vi "cycloid_text_file_generator.vi"() -> ()   [LabVIEW 2025]
panel:
  out "?":path
  out "cycle time triangle":dbl min=0.0 step=0.01
  out "Total # points triangle":i32 min=0 step=1
  out "Total Time triangle":dbl min=0.0 step=0.01
  out "Total time for one cycle Triangle":dbl min=0.0 step=0.01
  out "A3":dbl min=0.0 step=0.01
  out "f_rise":dbl min=0.0 step=0.01
  out "Trs":dbl min=0.0 step=0.01
  out "Instantaneous Flyback Time Sawtooth":dbl min=0.0 step=0.01
  out "cycle time sawtooth":dbl min=0.0 step=0.01
  out "Total Time sawtooth":dbl min=0.0 step=0.01
  out "Total # points sawtooth":i32 min=0 step=1
  in  "Number of cycles":i32=1
  in  "Sample rate":i32=5000
  out "Total time for one cycle Sawtooth":dbl min=0.0 step=0.01
  out "A0 Offset By Position Error":dbl min=0.0 step=0.01
  out "A1 Offset By Position Error":dbl min=0.0 step=0.01
  out "Position error":dbl min=0.0 step=0.01
  out "A2":dbl min=0.0 step=0.01
  out "W":dbl=28.0 min=0.0 step=0.01
  in  "T":dbl=0.01 min=0.0 step=0.001
  out "Tf":dbl=-0.44999999999999996 min=0.0 step=0.01
  in  "Tracking Delay":dbl=1e-05 min=0.0 step=1e-05
  out "A0":dbl
  in  "Cycloid selector":u16(ring) items=["Triangle", "Sawtooth"]
  in  "OK Button":bool
  in  "stop button":bool
  out "XY Graph":cluster{dbl[], dbl[]}(graph)
  out "Ts":dbl min=0.0 step=0.01
  out "W2":dbl
  out "A1":dbl
  in  "TrampCV":dbl=0.0008 min=0.0 step=1e-05
  in  "A":i32=2
  # "Cycloid Waveform Generator"
  # "A: Amplitude (peak-to-peak) of the waveform in degrees\n\nT: Total time period for one complete cycle (seconds)\n\nTrampCV: Time duration of the constant velocity ramp portion (seconds)\n\nTrackingDelay: Time delay between input command and actual output (seconds)\n\nsample_rate: Number of samples per second\n\nnum_points: Number of points per cycle \n\nnum_cycles: Number of complete cycles to generate (default 1)\n\nA0: Starting position of the rising ramp (-A / 2)\n\nA1: Ending position of the rising ramp (+A / 2)\n\nTs: Total settling time = 2 * TrackingDelay\n\nTrs: Time for each sine transition (after ramp and settling)\n\nW: Slope of the ramp portion (deg/sec) = A / TrampCV\n\nf_rise: Frequency of the sine transition = 1 / (2 * Trs)\n\nA3: Amplitude of sine transition based on ramp slope and frequency\n\nPositionError: Position offset due to the delay = W * TrackingDelay\n\nA1OffsetByPositionError: Adjusted final position of ramp, including error\n\nA0OffsetByPositionError: Adjusted starting position of ramp, including error\n\nTotalTimeForOneCycle: Duration of one full waveform cycle (ramp + sine + fall + sine)\n\ntotal_points: Total number of sample points = sample_rate × TotalTimeForOneCycle × num_cycles\n\ntime_array: Array of time values for the full waveform\n\ncommand_signal: Output waveform values initialized to zero\n\nTf: Flyback (retrace) time\n\nW2: Angular frequency of the cycloidal retrace \n\nA2: Flyback amplitude \n\nInstantaneousFlybackTime: Time into the flyback portion of the waveform"
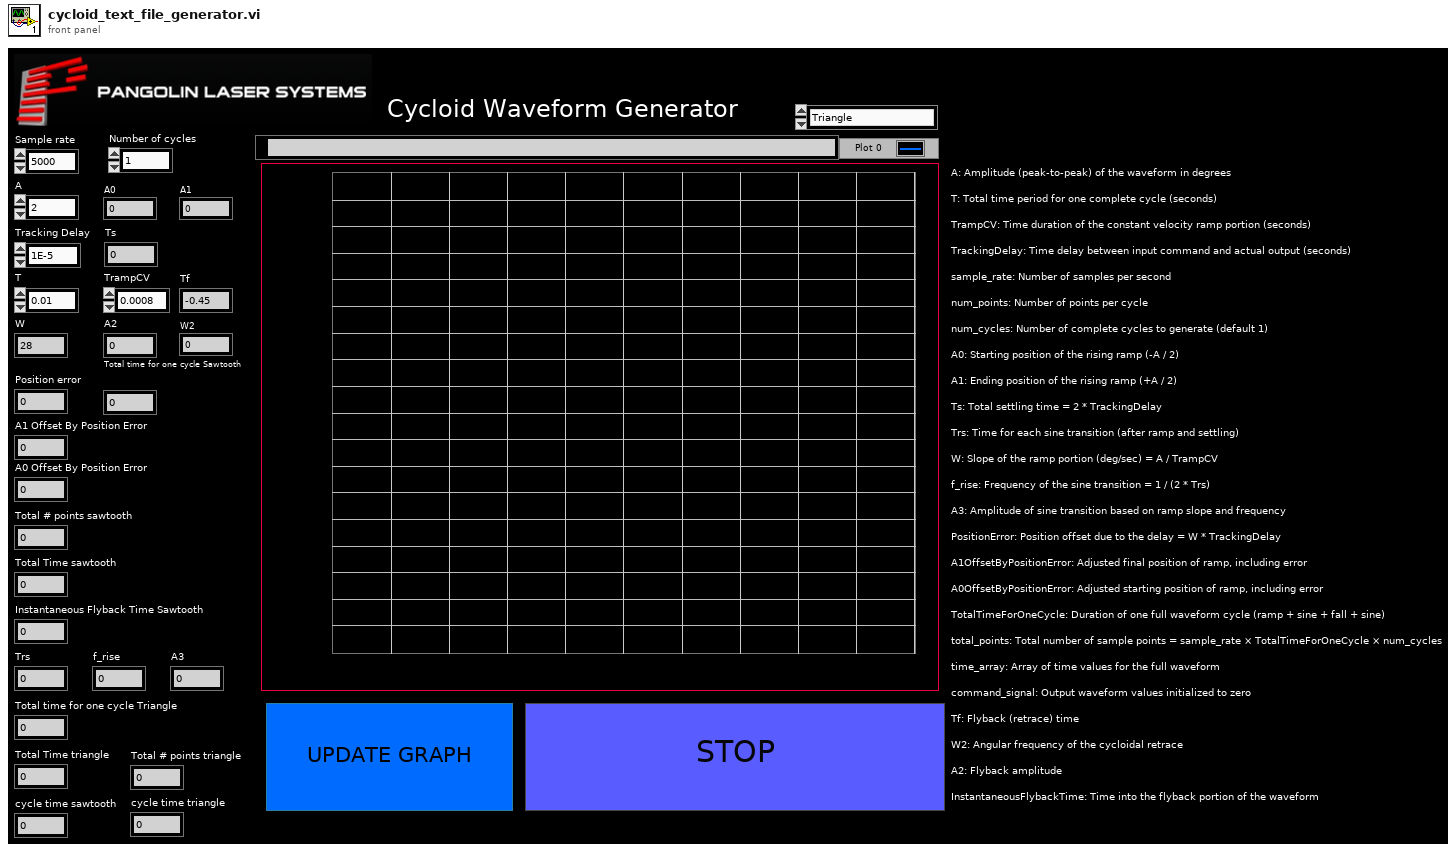
[diagram p1: front panel]
types:
  T1 = enum16{"open", "replace", "create", "open or create", "replace or create", "replace or create with confirmation"}
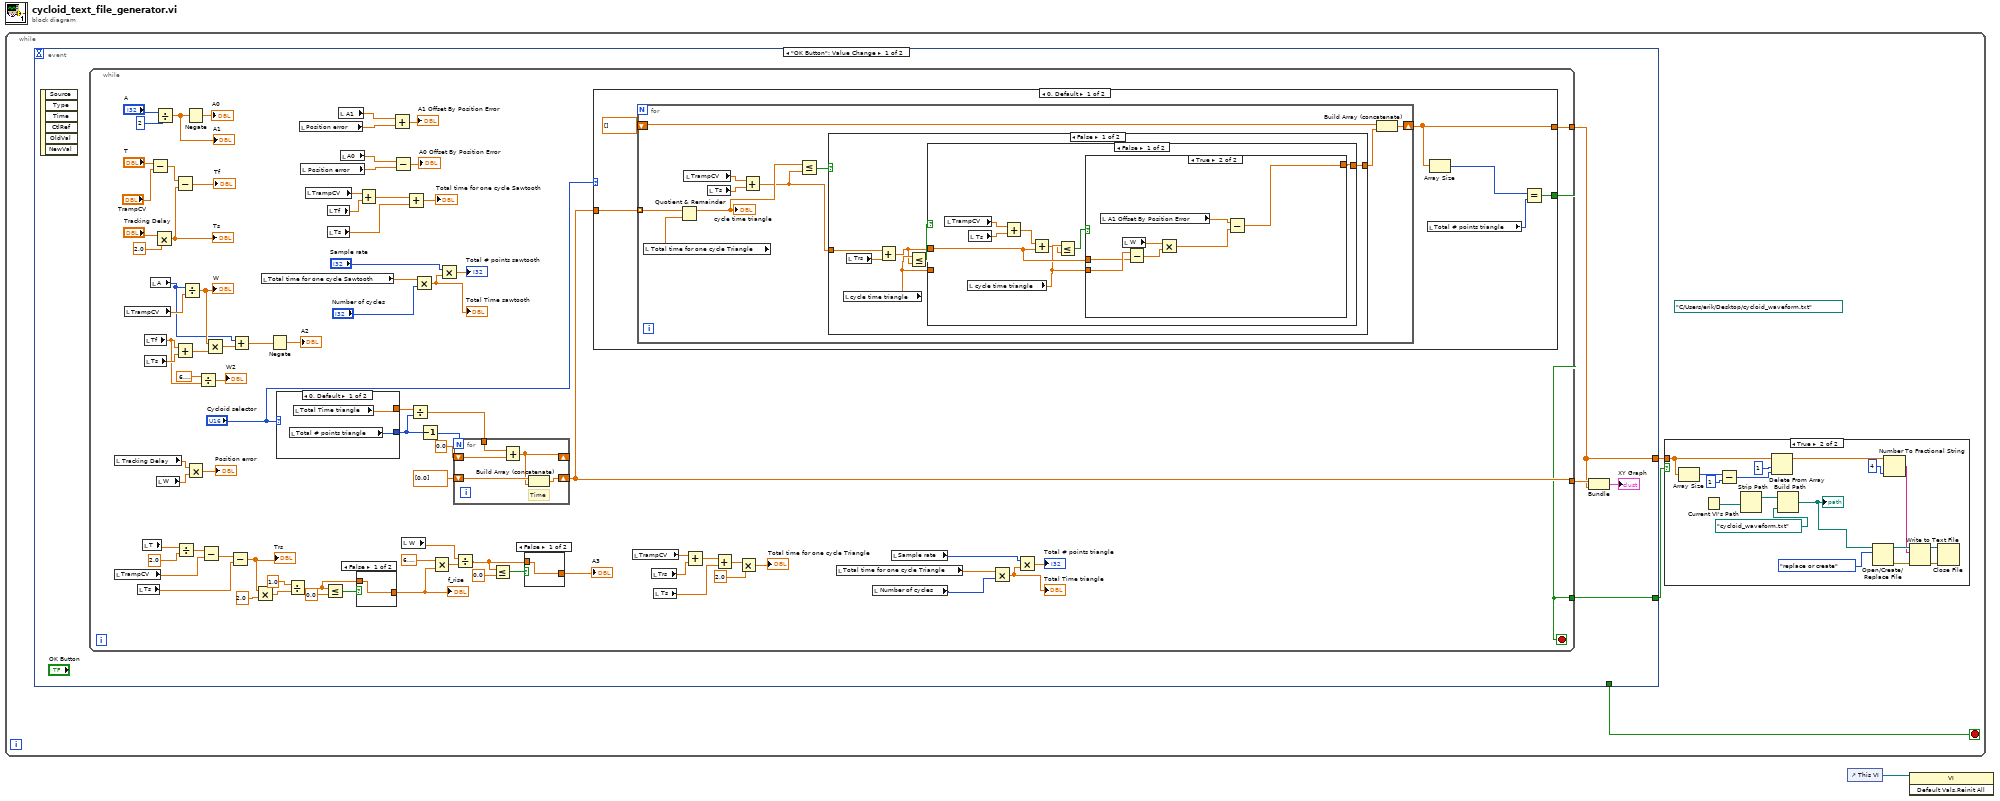
[diagram p0: block diagram]
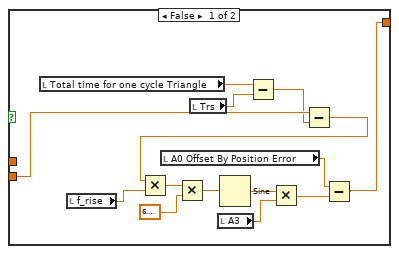
[diagram p3: hidden frame]
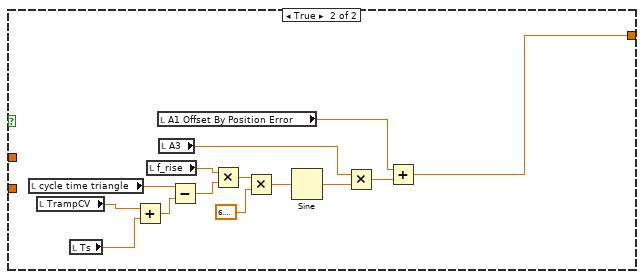
[diagram p4: hidden frame]
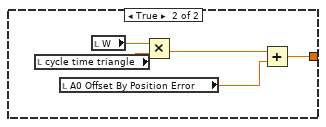
[diagram p5: hidden frame]
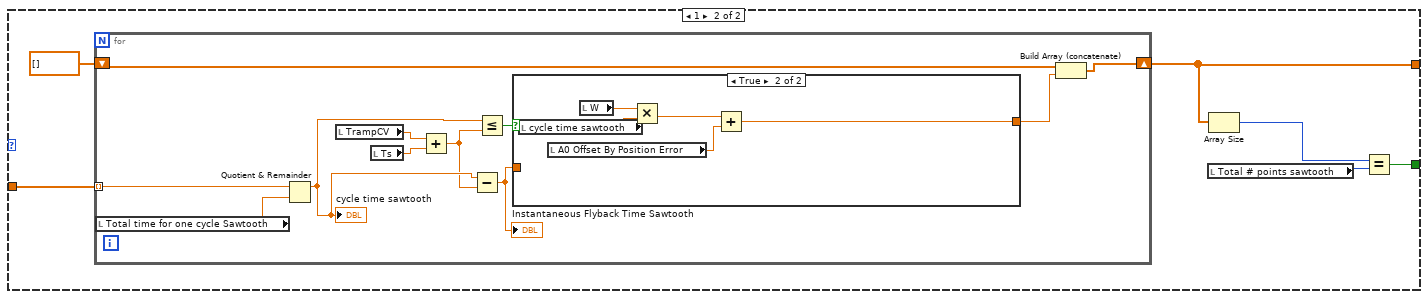
[diagram p6: hidden frame]
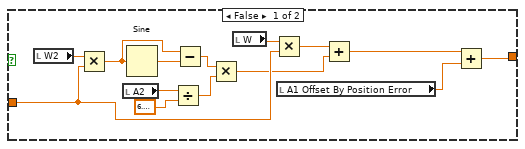
[diagram p7: hidden frame]
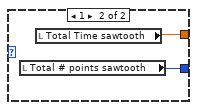
[diagram p8: hidden frame]
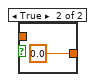
[diagram p9: hidden frame]
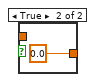
[diagram p10: hidden frame]
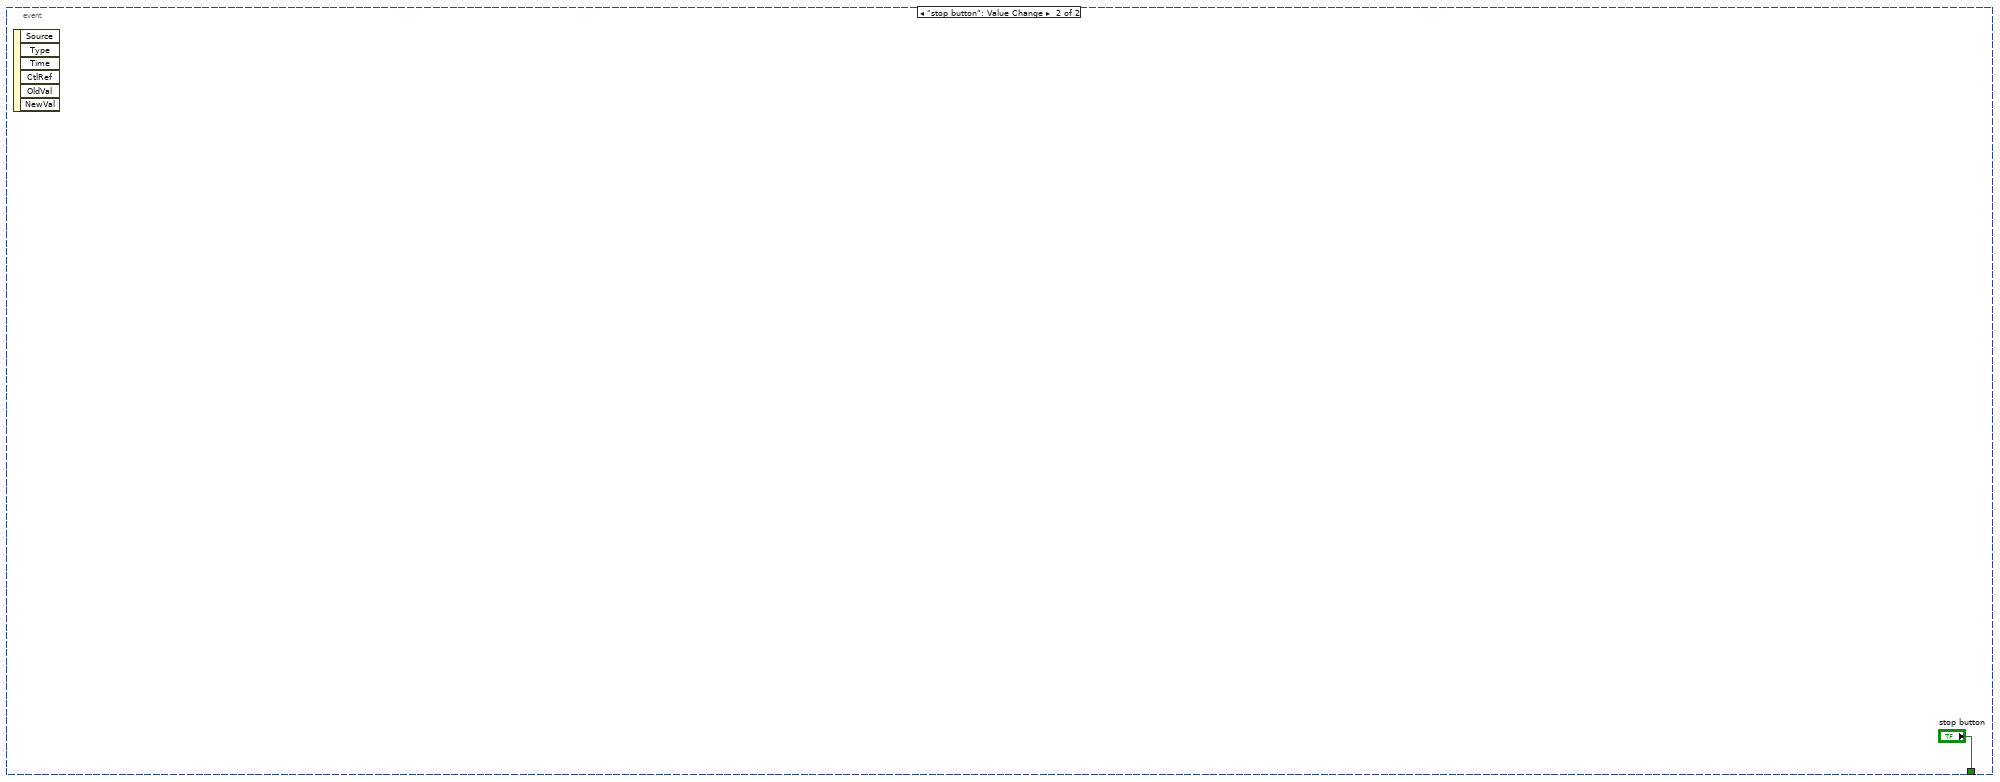
[diagram p11: hidden frame]
diagram:
  n1 = while {
    stop <- w3 stop-if-true
    (unwired) path "C:/Users/erik/Desktop/cycloid_waveform.txt" ("file path (use dialog)")
    n2 = event shown="[0] \"OK Button\": Value Change" {
      selector: _ -> [_ _]
      dyn-events: _ -> [_ _]
      timeout: _ -> [_ _]
      tunnel: [w24 _] -> w4
      tunnel: [_ "stop button"] -> w3
      tunnel: [w22 _] -> w2
      event "OK Button": Value Change {
        n3 = event-data() -> ()  [unwired: 1 in, 6 out]
        n4 = while {
          tunnel: [w62] -> w25
          tunnel: [w61] -> w24
          tunnel: [w26] -> w22
          stop <- w26 stop-if-true
          n5 = local read "TrampCV"() -> (w57:dbl)
          n6 = local read "Tracking Delay"() -> (w87:dbl)
          n7 = local read "TrampCV"() -> (w98:dbl)
          n8 = local read "Ts"() -> (w55:dbl)
          n9 = local read "T"() -> (w60:dbl)
          n10 = local read "Tf"() -> (w90:dbl)
          n11 = local read "Ts"() -> (w97:dbl)
          n12 = Subtract(x="T", y="TrampCV") -> (x-y=w101:dbl)
          n13 = local read "A"() -> (w93:i32)
          n14 = Multiply(x="Tracking Delay", y=2.0) -> (x*y=w99:dbl)
          "Ts" <- w99
          n15 = Divide(x="A", y=2) -> (x/y=w106:dbl)
          "A1" <- w106
          n16 = local read "W"() -> (w86:dbl)
          n17 = Subtract(x=w101, y=w99) -> (x-y=→"Tf":dbl)
          n18 = Add(x=w90, y=w97) -> (x+y=w96:dbl)
          n19 = Divide(x=w60, y=2.0) -> (x/y=w58:dbl)
          n20 = Divide(x=w93, y=w98) -> (x/y=w95:dbl)
          "W" <- w95
          n21 = Negate(x=w106) -> (-x=→"A0":dbl)
          n22 = Multiply(x=w87, y=w86) -> (x*y=→"Position error":dbl)
          n23 = Divide(x=6.283185307179586, y=w90) -> (x/y=→"W2":dbl)
          n24 = Subtract(x=w58, y=w57) -> (x-y=w56:dbl)
          n25 = Multiply(x=w95, y=w96) -> (x*y=w94:dbl)
          n26 = Subtract(x=w56, y=w55) -> (x-y=w27:dbl)
          "Trs" <- w27
          n27 = Add(x=w93, y=w94) -> (x+y=w92:dbl)
          n28 = Multiply(x=w27, y=2.0) -> (x*y=w53:dbl)
          n29 = local read "Total time for one cycle Sawtooth"() -> (w63:dbl)
          n30 = Negate(x=w92) -> (-x=→"A2":dbl)
          n31 = case shown="0, Default" "Cycloid selector" {
            tunnel: [w217 w219] -> w69
            tunnel: [w216 w218] -> w65
            frame 0, Default {
              n32 = local read "Total # points triangle"() -> (w216:i32)
              n33 = local read "Total Time triangle"() -> (w217:dbl)
            }
            frame 1 {
              n34 = local read "Total # points sawtooth"() -> (w218:i32)
              n35 = local read "Total Time sawtooth"() -> (w219:dbl)
            }
          }
          n36 = Divide(x=1.0, y=w53) -> (x/y=w49:dbl)
          n37 = local read "Position error"() -> (w83:dbl)
          n38 = local read "Position error"() -> (w80:dbl)
          n39 = local read "TrampCV"() -> (w78:dbl)
          n40 = Less Or Equal?(x=w49, y=0.0) -> (x <= y?=w50:bool)
          n41 = local read "Tf"() -> (w77:dbl)
          n42 = local read "Ts"() -> (w75:dbl)
          n43 = local read "A1"() -> (w84:dbl)
          n44 = local read "A0"() -> (w79:dbl)
          n45 = case shown="False" w50 {
            tunnel: [w222 0.0 ("y")] -> w48
            tunnel: w49 -> [w222 _]
            frame False {
            }
            frame True {
            }
          }
          "f_rise" <- w48
          n46 = Add(x=w78, y=w77) -> (x+y=w76:dbl)
          n47 = Add(x=w84, y=w83) -> (x+y=→"A1 Offset By Position Error":dbl)
          n48 = Subtract(x=w79, y=w80) -> (x-y=→"A0 Offset By Position Error":dbl)
          n49 = local read "W"() -> (w45:dbl)
          n50 = Add(x=w76, y=w75) -> (x+y=→"Total time for one cycle Sawtooth":dbl)
          n51 = Divide(x=w69, y=w65) -> (x/y=w68:dbl)
          n52 = Multiply(x=w63, y="Number of cycles") -> (x*y=w70:dbl)
          "Total Time sawtooth" <- w70
          n53 = Decrement(x=w65) -> (x-1=w64:i32)
          n54 = Multiply(x=6.283185307179586, y=w48) -> (x*y=w46:dbl)
          n55 = Multiply(x="Sample rate", y=w70) -> (x*y=→"Total # points sawtooth":dbl)
          n56 = for {
            N: w64 -> [_]
            shift-right: [w228] -> w62
            shift-left: dbl[] [0.0] -> [w227]
            tunnel: w68 -> [w225]
            shift-right: [w224] -> _
            shift-left: 0.0 -> [w226]
            # "Time"
            n57 = Add(x=w225, y=w226) -> (x+y=w224:dbl)
            n58 = Build Array (concatenate)(w227, w224) -> (w228:dbl[])
          }
          n59 = Divide(x=w45, y=w46) -> (x/y=w41:dbl)
          n60 = Less Or Equal?(x=w41, y=0.0) -> (x <= y?=w44:bool)
          n61 = case shown="False" w44 {
            tunnel: [w220 0.0 ("y")] -> w42
            tunnel: w41 -> [w220 _]
            frame False {
            }
            frame True {
            }
          }
          "A3" <- w42
          n62 = case shown="0, Default" "Cycloid selector" {
            tunnel: w62 -> [w112 w185]
            tunnel: [w113 w183] -> w61
            tunnel: [w110 w180] -> w26
            frame 0, Default {
              n63 = for {
                tunnel: w112 -> [w125] mode=indexing
                shift-right: [w122] -> w113
                shift-left: dbl[] [] -> [w121]
                n64 = local read "Total time for one cycle Triangle"() -> (w119:dbl)
                n65 = Quotient & Remainder(x=w125, y=w119) -> (x-y*floor(x/y)=w117:dbl)  [unwired: 1 out]
                "cycle time triangle" <- w117
                n66 = local read "TrampCV"() -> (w124:dbl)
                n67 = local read "Ts"() -> (w118:dbl)
                n68 = Add(x=w124, y=w118) -> (x+y=w116:dbl)
                n69 = Less Or Equal?(x=w117, y=w116) -> (x <= y?=w123:bool)
                n70 = case shown="False" w123 {
                  tunnel: [w128 w175] -> w120
                  tunnel: w116 -> [w130 _]
                  frame False {
                    n71 = local read "cycle time triangle"() -> (w127:dbl)
                    n72 = local read "Trs"() -> (w131:dbl)
                    n73 = Add(x=w130, y=w131) -> (x+y=w126:dbl)
                    n74 = Less Or Equal?(x=w127, y=w126) -> (x <= y?=w129:bool)
                    n75 = case shown="False" w129 {
                      tunnel: w127 -> [_ _]
                      tunnel: [w134 w162] -> w128
                      tunnel: w126 -> [w135 _]
                      frame False {
                        n76 = local read "TrampCV"() -> (w138:dbl)
                        n77 = local read "cycle time triangle"() -> (w133:dbl)
                        n78 = local read "Ts"() -> (w139:dbl)
                        n79 = Add(x=w138, y=w139) -> (x+y=w137:dbl)
                        n80 = Add(x=w137, y=w135) -> (x+y=w132:dbl)
                        n81 = Less Or Equal?(x=w133, y=w132) -> (x <= y?=w136:bool)
                        n82 = case shown="True" w136 {
                          tunnel: w133 -> [w151 w160]
                          tunnel: w135 -> [_ w159]
                          tunnel: [w140 w154] -> w134
                          frame False {
                            n83 = local read "Total time for one cycle Triangle"() -> (w153:dbl)
                            n84 = local read "f_rise"() -> (w149:dbl)
                            n85 = local read "A0 Offset By Position Error"() -> (w141:dbl)
                            n86 = local read "Trs"() -> (w152:dbl)
                            n87 = local read "A3"() -> (w144:dbl)
                            n88 = Subtract(x=w153, y=w152) -> (x-y=w150:dbl)
                            n89 = Subtract(x=w151, y=w150) -> (x-y=w148:dbl)
                            n90 = Multiply(x=w148, y=w149) -> (x*y=w142:dbl)
                            n91 = Multiply(x=w142, y=6.283185307179586) -> (x*y=w146:dbl)
                            n92 = Sine(x=w146) -> (sin(x)=w145:dbl)
                            n93 = Multiply(x=w145, y=w144) -> (x*y=w143:dbl)
                            n94 = Subtract(x=w141, y=w143) -> (x-y=w140:dbl)
                          }
                          frame True {
                            n95 = local read "A1 Offset By Position Error"() -> (w156:dbl)
                            n96 = local read "W"() -> (w157:dbl)
                            n97 = Subtract(x=w160, y=w159) -> (x-y=w158:dbl)
                            n98 = Multiply(x=w157, y=w158) -> (x*y=w155:dbl)
                            n99 = Subtract(x=w156, y=w155) -> (x-y=w154:dbl)
                          }
                        }
                      }
                      frame True {
                        n100 = local read "cycle time triangle"() -> (w161:dbl)
                        n101 = local read "TrampCV"() -> (w174:dbl)
                        n102 = local read "Ts"() -> (w173:dbl)
                        n103 = Add(x=w174, y=w173) -> (x+y=w172:dbl)
                        n104 = local read "f_rise"() -> (w171:dbl)
                        n105 = local read "A1 Offset By Position Error"() -> (w163:dbl)
                        n106 = local read "A3"() -> (w165:dbl)
                        n107 = Subtract(x=w161, y=w172) -> (x-y=w170:dbl)
                        n108 = Multiply(x=w171, y=w170) -> (x*y=w169:dbl)
                        n109 = Multiply(x=w169, y=6.283185307179586) -> (x*y=w167:dbl)
                        n110 = Sine(x=w167) -> (sin(x)=w166:dbl)
                        n111 = Multiply(x=w165, y=w166) -> (x*y=w164:dbl)
                        n112 = Add(x=w163, y=w164) -> (x+y=w162:dbl)
                      }
                    }
                  }
                  frame True {
                    n113 = local read "cycle time triangle"() -> (w178:dbl)
                    n114 = local read "A0 Offset By Position Error"() -> (w176:dbl)
                    n115 = local read "W"() -> (w179:dbl)
                    n116 = Multiply(x=w179, y=w178) -> (x*y=w177:dbl)
                    n117 = Add(x=w177, y=w176) -> (x+y=w175:dbl)
                  }
                }
                n118 = Build Array (concatenate)(w121, w120) -> (w122:dbl[])
              }
              n119 = local read "Total # points triangle"() -> (w111:i32)
              n120 = Array Size(array=w113) -> (size(s)=w115:i32)
              n121 = Equal?(x=w115, y=w111) -> (x = y?=w110:bool)
            }
            frame 1 {
              n122 = for {
                tunnel: w185 -> [w195] mode=indexing
                shift-right: [w191] -> w183
                shift-left: dbl[] [] -> [w190]
                n123 = local read "Total time for one cycle Sawtooth"() -> (w196:dbl)
                n124 = Quotient & Remainder(x=w195, y=w196) -> (x-y*floor(x/y)=w188:dbl)  [unwired: 1 out]
                "cycle time sawtooth" <- w188
                n125 = local read "TrampCV"() -> (w194:dbl)
                n126 = local read "Ts"() -> (w193:dbl)
                n127 = Add(x=w194, y=w193) -> (x+y=w187:dbl)
                n128 = Subtract(x=w188, y=w187) -> (x-y=w186:dbl)
                "Instantaneous Flyback Time Sawtooth" <- w186
                n129 = Less Or Equal?(x=w188, y=w187) -> (x <= y?=w192:bool)
                n130 = case shown="True" w192 {
                  tunnel: [w198 w211] -> w189
                  tunnel: w186 -> [w202 _]
                  frame False {
                    n131 = local read "W2"() -> (w210:dbl)
                    n132 = Multiply(x=w210, y=w202) -> (x*y=w208:dbl)
                    n133 = local read "A2"() -> (w207:dbl)
                    n134 = Sine(x=w208) -> (sin(x)=w209:dbl)
                    n135 = Divide(x=w207, y=6.283185307179586) -> (x/y=w204:dbl)
                    n136 = Subtract(x=w208, y=w209) -> (x-y=w205:dbl)
                    n137 = Multiply(x=w205, y=w204) -> (x*y=w200:dbl)
                    n138 = local read "W"() -> (w203:dbl)
                    n139 = Multiply(x=w203, y=w202) -> (x*y=w201:dbl)
                    n140 = local read "A1 Offset By Position Error"() -> (w197:dbl)
                    n141 = Add(x=w201, y=w200) -> (x+y=w199:dbl)
                    n142 = Add(x=w199, y=w197) -> (x+y=w198:dbl)
                  }
                  frame True {
                    n143 = local read "cycle time sawtooth"() -> (w214:dbl)
                    n144 = local read "A0 Offset By Position Error"() -> (w212:dbl)
                    n145 = local read "W"() -> (w215:dbl)
                    n146 = Multiply(x=w215, y=w214) -> (x*y=w213:dbl)
                    n147 = Add(x=w213, y=w212) -> (x+y=w211:dbl)
                  }
                }
                n148 = Build Array (concatenate)(w190, w189) -> (w191:dbl[])
              }
              n149 = local read "Total # points sawtooth"() -> (w181:i32)
              n150 = Array Size(array=w183) -> (size(s)=w182:i32)
              n151 = Equal?(x=w182, y=w181) -> (x = y?=w180:bool)
            }
          }
          n152 = local read "TrampCV"() -> (w38:dbl)
          n153 = local read "Trs"() -> (w37:dbl)
          n154 = local read "Ts"() -> (w40:dbl)
          n155 = Add(x=w38, y=w37) -> (x+y=w39:dbl)
          n156 = Add(x=w39, y=w40) -> (x+y=w36:dbl)
          n157 = Multiply(x=w36, y=2.0) -> (x*y=→"Total time for one cycle Triangle":dbl)
          n158 = local read "Total time for one cycle Triangle"() -> (w30:dbl)
          n159 = local read "Number of cycles"() -> (w29:i32)
          n160 = local read "Sample rate"() -> (w31:i32)
          n161 = Multiply(x=w30, y=w29) -> (x*y=w33:dbl)
          "Total Time triangle" <- w33
          n162 = Multiply(x=w31, y=w33) -> (x*y=→"Total # points triangle":dbl)
        }
        n163 = Bundle(w25, w24) -> (→"XY Graph":cluster{dbl[], dbl[]})  [unwired: 1 in]
      }
      event "stop button": Value Change {
        n164 = event-data() -> ()  [unwired: 1 in, 6 out]
      }
    }
    n165 = case shown="True" w2 {
      tunnel: w4 -> [_ w21]
      frame False {
      }
      frame True {
        n166 = Array Size(array=w21) -> (size(s)=w12:i32)
        n167 = Current VI's Path() -> (path=w7:path)
        n168 = Subtract(x=w12, y=1) -> (x-y=w10:i32)
        n169 = Strip Path(path=w7) -> (stripped path=w8:path)  [unwired: 1 out]
        n170 = Delete From Array(array=w21, length=1, index=w10) -> (array with subset deleted=w15:dbl[])  [unwired: 1 out]
        n171 = Build Path(base path=w8, name or relative path=path "cycloid_waveform.txt") -> (appended path=w5:path)
        "?" <- w5
        n172 = Open/Create/Replace File(file path (use dialog)=w5, operation (0:open)=T1."replace or create") -> (refnum out=w20:refnum<file>, error out=w19:errorcluster)  [unwired: 4 in, 1 out]
        n173 = Number To Fractional String(number=w15, precision (6)=i16 4 ("width (-)")) -> (F-format string=w16:string[])  [unwired: 2 in]
        n174 = Write to Text File(file (use dialog)=w20, text=w16, error in=w19) -> (refnum out=w18:refnum<file>, error out=w17:errorcluster)  [unwired: 1 in, 1 out]
        n175 = Close File(refnum=w18, error in=w17) -> ()  [unwired: 2 out]
      }
    }
  }
  n176 = control-ref of="This VI"() -> (w1:refnum<vi>)
  n177 = invoke class="VI" method="Default Vals.Reinit All"(reference=w1) -> ()  [unwired: 2 in, 3 out]
